vi "Shooter BEGIN.vi"   [LabVIEW 2016]
uses:
  <vilib>/Rock Robotics/WPI/ThirdParty/CanMotor/TalonSRX/WPI_CANTalonSRX_APIControlMode.ctl
  <vilib>/Rock Robotics/WPI/ThirdParty/CanMotor/TalonSRX/WPI_CANTalonSRX_BrakeOverride.ctl
  <vilib>/Rock Robotics/WPI/ThirdParty/CanMotor/TalonSRX/WPI_CANTalonSRX_APIFeedbackSelect.ctl
  <vilib>/Rock Robotics/WPI/SafetyOutput/WPI_SafetyOutputConfigMenu.ctl
  Robot Global Data.vi
types:
  T1 = typedef "WPI_SafetyOutputConfigMenu.ctl" = enum16{"Enable", "Disable"}
  T2 = typedef "WPI_CANTalonSRX_APIFeedbackSelect.ctl" = enum16{"Digital Quadrature Encoder", "Analog Potentiometer", "Analog Encoder", "Count on Quad-A (Rising-Edge)", "Count on Quad-A (Falling-Edge)", "CTR Magnetic Enc (Absolute)", "CTR Magnetic Enc (Relative)", "Pulse Width"}
  T3 = typedef "WPI_CANTalonSRX_BrakeOverride.ctl" = enum8{"No Override", "Override to Coast", "Override to Brake"}
  T4 = typedef "WPI_CANTalonSRX_APIControlMode.ctl" = enum8{"Percent VBus", "Speed", "Position", "Slave", "Unchanged / Invalid", "Voltage Compensation", "Current", "Motion Profile", "Motion Magic"}
  T5 = typedef "WPI_MotorControlDeviceRef.ctl" = cluster{"DeviceStatus":errorcluster, "Type":T6, "PWM":cluster{"PWM Channel":T7, "DeadBand":T8}, "CAN":cluster{"Device Number":u8, "SetOutput VI Ref":variant, "GetOutput VI Ref":variant, "Enable VI Ref":variant, "Disable VI Ref":variant, "Data":variant}, "Invert":bool}
  T6 = typedef "WPI_MotorControlType.ctl" = enum16{"PWM", "CAN"}
  T7 = typedef "FPGA_DIOPWMChannel.ctl" = enum8{"PWM 0", "PWM 1", "PWM 2", "PWM 3", "PWM 4", "PWM 5", "PWM 6", "PWM 7", "PWM 8", "PWM 9", "PWM MXP 0", "PWM MXP 1", "PWM MXP 2", "PWM MXP 3", "PWM MXP 4", "PWM MXP 5", "PWM MXP 6", "PWM MXP 7", "PWM MXP 8", "PWM MXP 9", "Invalid"}
  T8 = typedef "WPI_PWMDeadband.ctl" = cluster{"Name":string, "maxPositivePwm":i32, "minPositivePwm":i32, "centerPwm":i32, "maxNegativePwm":i32, "minNegativePwm":i32, "angularRange":u16}
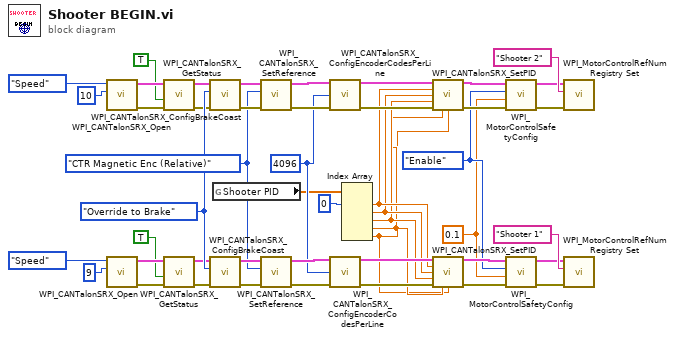
[diagram p0: block diagram]
diagram:
  w11 = WPI_SafetyOutputConfigMenu."Enable" ("mode")
  w10 = 0.1 ("timeout (s)")
  w32 = u32 4096 ("Number Encoder Lines\n(Counts Per Rotation)")
  w39 = WPI_CANTalonSRX_APIFeedbackSelect."CTR Magnetic Enc (Relative)" ("Feedback Reference")
  w44 = WPI_CANTalonSRX_BrakeOverride."Override to Brake" ("Brake / Coast Mode")
  n1 = call <vilib>:"WPI_CANTalonSRX_Open.vi"("Device Number"=u8 10, "Control Mode"=WPI_CANTalonSRX_APIControlMode."Speed") -> ("error out"=w31:errorcluster, "CAN Talon SRX Ref"=w30:T5)  [unwired: 8 in]
  n2 = call <vilib>:"WPI_CANTalonSRX_Open.vi"("Device Number"=u8 9, "Control Mode"=WPI_CANTalonSRX_APIControlMode."Speed") -> ("error out"=w25:errorcluster, "CAN Talon SRX Ref"=w26:T5)  [unwired: 8 in]
  n3 = call <vilib>:"WPI_CANTalonSRX_GetStatus.vi"("error in (no error)"=w31, "Clear Sticky Faults"=TRUE, "CAN Talon SRX Ref"=w30) -> ("error out"=w28:errorcluster, "CAN Talon SRX Ref"=w29:T5)  [unwired: 6 in, 1 out]
  n4 = call <vilib>:"WPI_CANTalonSRX_GetStatus.vi"("error in (no error)"=w25, "Clear Sticky Faults"=TRUE, "CAN Talon SRX Ref"=w26) -> ("error out"=w23:errorcluster, "CAN Talon SRX Ref"=w24:T5)  [unwired: 6 in, 1 out]
  n5 = call <vilib>:"WPI_CANTalonSRX_ConfigBrakeCoast.vi"("error in (no error)"=w28, "Brake / Coast Mode"=w44, "CAN Talon SRX Ref"=w29) -> ("error out"=w40:errorcluster, "CAN Talon SRX Ref"=w41:T5)  [unwired: 7 in]
  n6 = call <vilib>:"WPI_CANTalonSRX_ConfigBrakeCoast.vi"("error in (no error)"=w23, "Brake / Coast Mode"=w44, "CAN Talon SRX Ref"=w24) -> ("error out"=w42:errorcluster, "CAN Talon SRX Ref"=w43:T5)  [unwired: 7 in]
  n7 = global read "Robot Global Data.vi" "Shooter PID"() -> (w7:dbl[])
  n8 = call <vilib>:"WPI_CANTalonSRX_SetReference.vi"("error in (no error)"=w40, "Feedback Reference"=w39, "CAN Talon SRX Ref"=w41) -> ("error out"=w35:errorcluster, "CAN Talon SRX Ref"=w36:T5)  [unwired: 7 in]
  n9 = call <vilib>:"WPI_CANTalonSRX_SetReference.vi"("error in (no error)"=w42, "Feedback Reference"=w39, "CAN Talon SRX Ref"=w43) -> ("error out"=w37:errorcluster, "CAN Talon SRX Ref"=w38:T5)  [unwired: 7 in]
  n10 = call <vilib>:"WPI_CANTalonSRX_ConfigEncoderCodesPerLine.vi"("CAN Talon SRX Ref"=w36, "Number Encoder Lines\n(Counts Per Rotation)"=w32, "error in (no error)"=w35) -> ("CAN Talon SRX Ref"=w19:T5, "error out"=w18:errorcluster)  [unwired: 11 in]
  n11 = call <vilib>:"WPI_CANTalonSRX_ConfigEncoderCodesPerLine.vi"("CAN Talon SRX Ref"=w38, "Number Encoder Lines\n(Counts Per Rotation)"=w32, "error in (no error)"=w37) -> ("CAN Talon SRX Ref"=w20:T5, "error out"=w21:errorcluster)  [unwired: 11 in]
  n12 = Index Array(array=w7, index #1=0 ("index")) -> (element #1=w5:dbl, element #2=w4:dbl, element #3=w3:dbl, element #4=w2:dbl, element #5=w1:dbl)  [unwired: 4 in]
  n13 = call <vilib>:"WPI_CANTalonSRX_SetPID.vi"("CAN Talon SRX Ref"=w19, "P"=w5, "I"=w4, "D"=w3, "error in (no error)"=w18, "F"=w2, "I Zone"=w1) -> ("CAN Talon SRX Ref"=w17:T5, "error out"=w16:errorcluster)  [unwired: 7 in]
  n14 = call <vilib>:"WPI_CANTalonSRX_SetPID.vi"("CAN Talon SRX Ref"=w20, "P"=w5, "I"=w4, "D"=w3, "error in (no error)"=w21, "F"=w2, "I Zone"=w1) -> ("CAN Talon SRX Ref"=w13:T5, "error out"=w12:errorcluster)  [unwired: 7 in]
  n15 = call <vilib>:"WPI_MotorControlSafetyConfig.vi"("error in (no error)"=w16, "timeout (s)"=w10, "mode"=w11, "MotorControlDevRef"=w17) -> ("error out"=w14:errorcluster, "MotorControlDevRef"=w15:T5)  [unwired: 6 in]
  n16 = call <vilib>:"WPI_MotorControlSafetyConfig.vi"("error in (no error)"=w12, "timeout (s)"=w10, "mode"=w11, "MotorControlDevRef"=w13) -> ("error out"=w8:errorcluster, "MotorControlDevRef"=w9:T5)  [unwired: 6 in]
  n17 = call <vilib>:"WPI_MotorControlRefNum Registry Set.vi"("error in (no error)"=w14, "refnum name"="Shooter 2", "MotorControlDevRef"=w15) -> ()  [unwired: 7 in, 2 out]
  n18 = call <vilib>:"WPI_MotorControlRefNum Registry Set.vi"("error in (no error)"=w8, "refnum name"="Shooter 1", "MotorControlDevRef"=w9) -> ()  [unwired: 7 in, 2 out]
